vi "send stop.vi"(8 "error in (no error)":errorcluster) -> (0 "error out":errorcluster)   [LabVIEW 2020, in "ui-testing.lvlib"]
uses:
  ui-testing.lvlib
  <vilib>/addons/zeromq/socket_type.ctl
  message.ctl
  <vilib>/addons/zeromq/zmq_context.lvclass
  <vilib>/addons/zeromq/zeromq.lvlib
  <vilib>/addons/zeromq/zmq_socket.lvclass
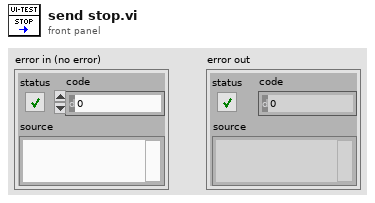
[diagram p1: front panel]
types:
  T1 = typedef "ui-testing.lvlib/message.ctl" = cluster{"message":string, "payload":string}
  T2 = typedef "zeromq.lvlib/socket_type.ctl" = enum8{"ZMQ_PAIR", "ZMQ_PUB", "ZMQ_SUB", "ZMQ_REQ", "ZMQ_REP", "ZMQ_DEALER", "ZMQ_ROUTER", "ZMQ_PULL", "ZMQ_PUSH", "ZMQ_XPUB", "ZMQ_XSUB", "ZMQ_STREAM", "ZMQ_SERVER", "ZMQ_CLIENT", "ZMQ_RADIO", "ZMQ_DISH", "ZMQ_GATHER", "ZMQ_SCATTER", "ZMQ_DGRAM"}
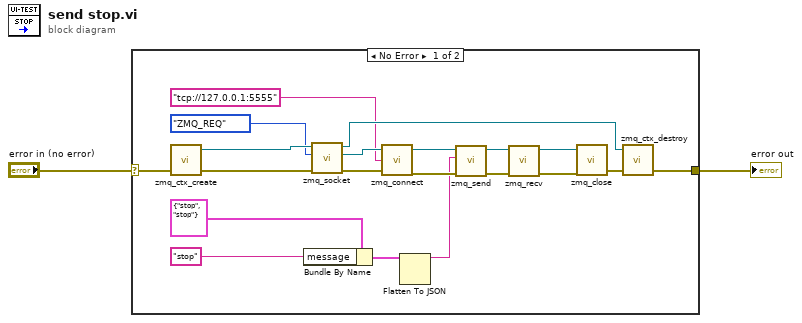
[diagram p0: block diagram]
diagram:
  n1 = case shown="No Error" "error in (no error)" {
    selector: "error in (no error)" -> [w3 w23]
    tunnel: [w4 w23] -> w2
    frame No Error {
      n2 = call <vilib>:"zmq_ctx_create.vi"("error in"=w3) -> ("error out"=w16:errorcluster, "context out"=w15:refnum<class "zmq_context.lvclass">)  [unwired: 3 in]
      n3 = Bundle By Name(cluster=T1 {"message"="stop", "payload"="stop"}, "message"="stop" ("data")) -> (w6:T1)
      n4 = call <vilib>:"zmq_socket.vi"("error in"=w16, "socket type"=socket_type."ZMQ_REQ", "context in"=w15) -> ("error out"=w18:errorcluster, "socket out"=w17:refnum<class "zmq_socket.lvclass">, "context out"=w22:refnum<class "zmq_context.lvclass">)  [unwired: 2 in]
      n5 = call <vilib>:"zmq_connect.vi"("error in"=w18, "endpoint"="tcp://127.0.0.1:5555", "socket in"=w17) -> ("error out"=w20:errorcluster, "socket out"=w19:refnum<class "zmq_socket.lvclass">)  [unwired: 1 in]
      n6 = Flatten To JSON(anything=w6) -> (JSON string=w7:string)  [unwired: 2 in, 1 out]
      n7 = call <vilib>:"zmq_send.vi"("error in"=w20, "data"=w7, "socket in"=w19) -> ("error out"=w11:errorcluster, "socket out"=w12:refnum<class "zmq_socket.lvclass">)  [unwired: 4 in]
      n8 = call <vilib>:"zmq_recv.vi"("error in"=w11, "socket in"=w12) -> ("error out"=w9:errorcluster, "socket out"=w10:refnum<class "zmq_socket.lvclass">)  [unwired: 3 in, 3 out]
      n9 = call <vilib>:"zmq_close.vi"("error in"=w9, "socket"=w10) -> ("error out"=w21:errorcluster)  [unwired: 3 in]
      n10 = call <vilib>:"zmq_ctx_destroy.vi"("error in"=w21, "context in"=w22) -> ("error out"=w4:errorcluster)  [unwired: 3 in]
    }
    frame Error {
    }
  }
  "error out" <- w2
